vi "Register All Controls.vi"(8 "error in (no error)":errorcluster, 10 "VI Refnum":refnum<vi>, 11 "ATM View Model in":refnum<class "ATM View Model.lvclass">) -> (0 "error out":errorcluster, 3 "ATM View Model out":refnum<class "ATM View Model.lvclass">)   [LabVIEW 2020, in "ATM View Model.lvclass"]
uses:
  ATM View Model.lvclass
  Controls.ctl
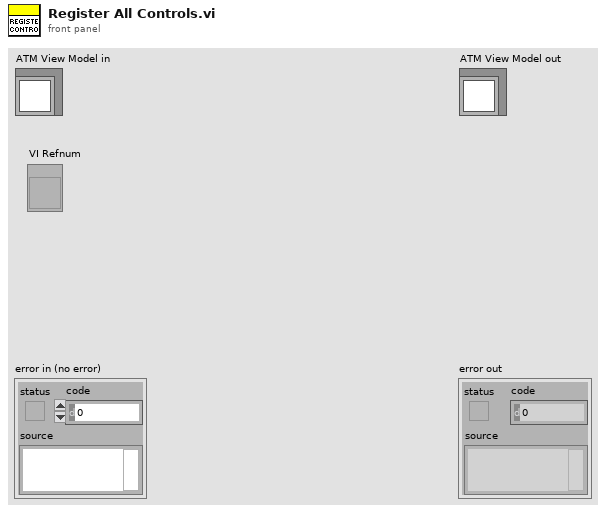
[diagram p1: front panel]
types:
  T1 = typedef "ATM View Model.lvclass/Controls.ctl" = enum16{"User Input", "Enter", "Left Menu", "Right Menu", "Left Button", "Right Button", "Card Simulator"}
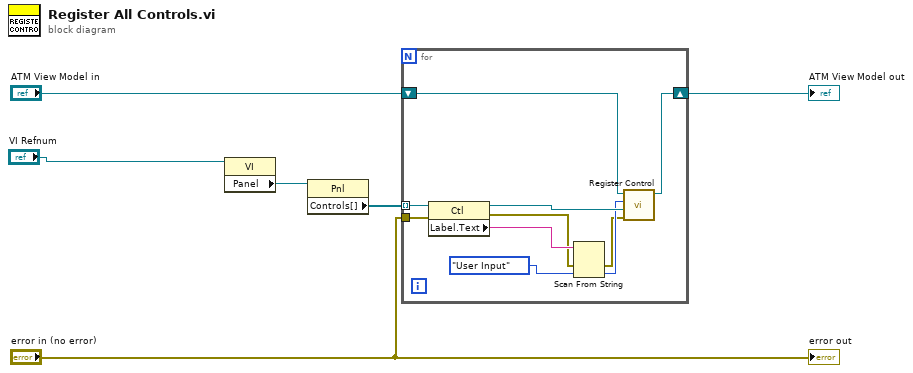
[diagram p0: block diagram]
diagram:
  n1 = property class="VI"(reference="VI Refnum") -> ("Panel"=w5:refnum<vi>)  [unwired: 1 in, 2 out]
  n2 = property class="Pnl"(reference=w5) -> ("Controls[]"=w4:refnum<vi>[])  [unwired: 1 in, 2 out]
  n3 = for {
    tunnel: w4 -> [w16] mode=indexing
    shift-right: [w14] -> w2
    shift-left: "ATM View Model in" -> [w15]
    tunnel: "error in (no error)" -> [w13]
    n4 = property class="Ctl"(reference=w16, error in=w13) -> (reference out=w12:refnum<vi>, error out=w7:errorcluster, "Label.Text"=w11:string)
    n5 = Scan From String(input string=w11, error in=w7, default 1=Controls."User Input" ("Control")) -> (error out=w8:errorcluster, output 1=w9:T1)  [unwired: 2 in, 2 out]
    n6 = call "Register Control.vi"("error in (no error)"=w8, "Control ref"=w12, "Control"=w9, "ATM View Model in"=w15) -> ("ATM View Model out"=w14:refnum<class "ATM View Model.lvclass">)  [unwired: 6 in, 1 out]
  }
  "ATM View Model out" <- w2
  "error out" <- "error in (no error)"
